vi "ISEG_HVBoardGUI.NofChToByte.vi"(3 "NofCh":i32) -> (17 "Byte":dbl)   [LabVIEW 2014, in "ISEG_HVBoardGUI.lvlib"]
doc: "converts the channel number so in a number as a byte array as many posts as channel"
uses:
  ISEG_HVBoardGUI.lvlib
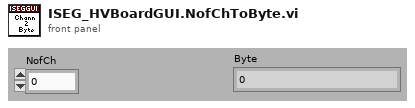
[diagram p1: front panel]
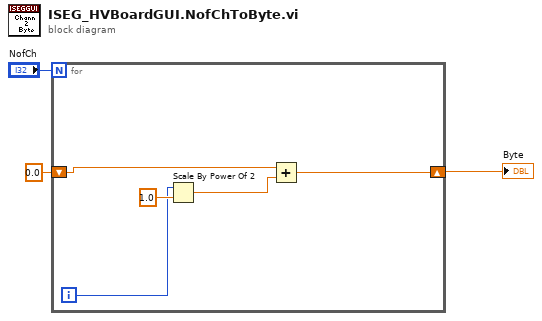
[diagram p0: block diagram]
diagram:
  n1 = for {
    N: "NofCh" -> [_]
    shift-right: [w6] -> w1
    shift-left: 0.0 -> [w7]
    i -> [w5]
    n2 = Scale By Power Of 2(n=w5, x=1.0) -> (x*2^n=w4:dbl)
    n3 = Add(x=w7, y=w4) -> (x+y=w6:dbl)
  }
  "Byte" <- w1
